vi "Change Voltage.vi"(8 "error in (no error)":errorcluster, 11 "Test Framework in":refnum<class "Test Framework.lvclass">) -> (0 "error out":errorcluster, 2 "PSU status":T1(array[cluster]), 3 "Test Framework out":refnum<class "Test Framework.lvclass">)   [LabVIEW 2020, in "Test Framework.lvclass"]
uses:
  Test Framework.lvclass
  Test Framework.lvclass/Test Framework.ctl
  Instruments/Power Supply/Power Supply.lvclass
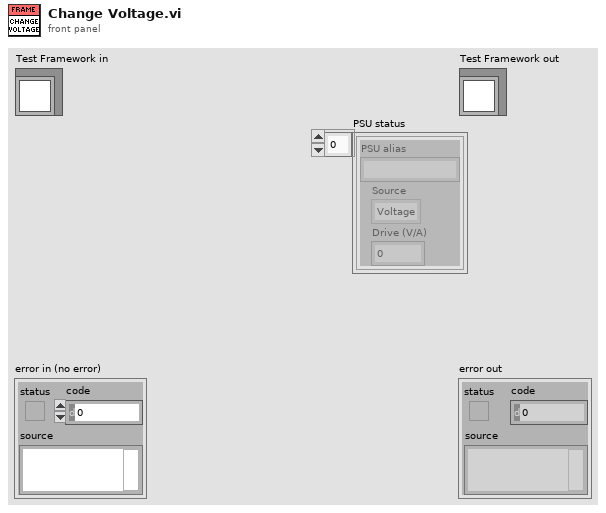
[diagram p1: front panel]
types:
  T1 = cluster{"PSU alias":string, "Source":enum32{"Voltage", "Current"}, "Drive (V/A)":dbl}[]
  T2 = cluster{"PSU alias":string, "Source":enum32{"Voltage", "Current"}, "Drive (V/A)":dbl}
  T3 = typedef "Test Framework.lvclass/Temperature and voltage array.ctl" = cluster{"Temperature [C]":dbl, "Soak time [m]":dbl, "PSUs":cluster{"Enabled":bool, "Source":enum32{"Voltage", "Current"}, "Drive (V/A)":dbl, "Sweep (V/A)":string, "Limit (A/V)":dbl, "PSU alias":string, "PSU info":cluster{"ID":string, "Address":string, "Channel":u8}}[]}[]
  T4 = typedef "Test Framework.lvclass/Temperature and voltage modes.ctl" = cluster{"Temperature mode":enum16{"Automatic", "Manual", "Off"}, "DC-Power mode":enum16{"Automatic", "Manual", "Off"}, "PSU sweep mode":bool, "Turn off after measurement":bool}
  T5 = cluster{"Temperature control array":T3, "Temperature mode":T4}
  T6 = cluster{"Temperature [C]":dbl, "Soak time [m]":dbl, "PSUs":cluster{"Enabled":bool, "Source":enum32{"Voltage", "Current"}, "Drive (V/A)":dbl, "Sweep (V/A)":string, "Limit (A/V)":dbl, "PSU alias":string, "PSU info":cluster{"ID":string, "Address":string, "Channel":u8}}[]}
  T7 = cluster{"Enabled":bool, "Source":enum32{"Voltage", "Current"}, "Drive (V/A)":dbl, "Sweep (V/A)":string, "Limit (A/V)":dbl, "PSU alias":string, "PSU info":cluster{"ID":string, "Address":string, "Channel":u8}}[]
  T8 = cluster{"ID":string, "Address":string, "Channel":u8}
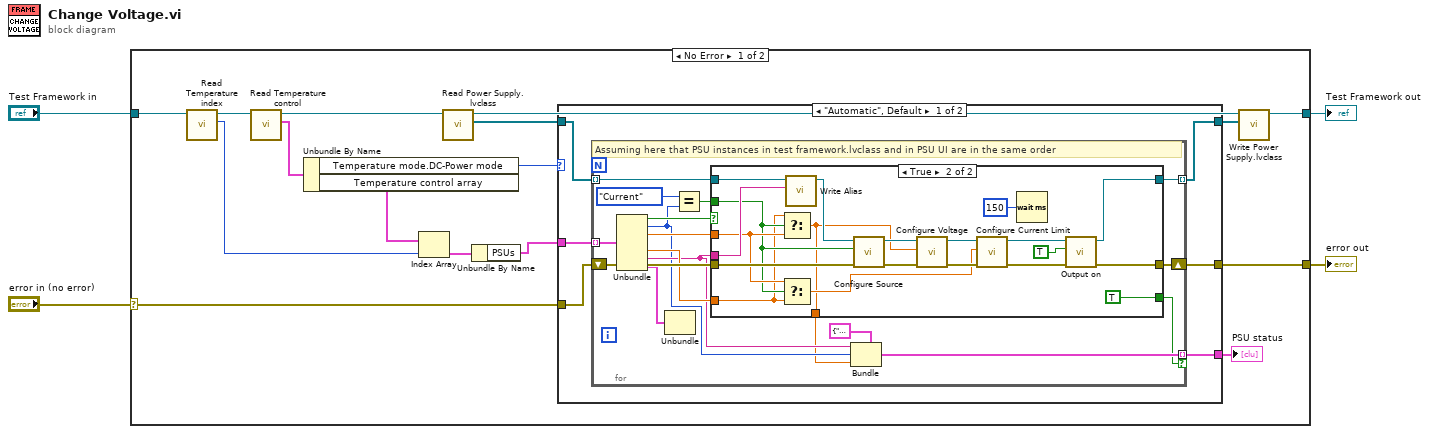
[diagram p0: block diagram]
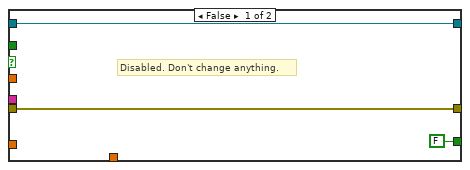
[diagram p2: hidden frame]
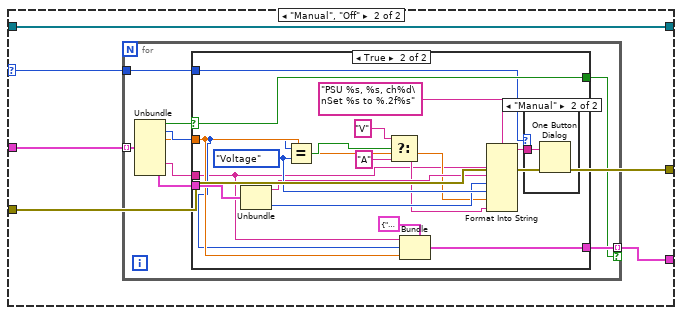
[diagram p3: hidden frame]
diagram:
  n1 = case shown="No Error" "error in (no error)" {
    selector: "error in (no error)" -> [w7 w100]
    tunnel: [w11 w100] -> w3
    tunnel: [w12 w99] -> w1
    tunnel: "Test Framework in" -> [w20 w99]
    frame No Error {
      n2 = call "Read Temperature index.vi"("Test Framework in"=w20) -> ("Environmental index"=w15:i32, "Test Framework out"=w19:refnum<class "Test Framework.lvclass">)  [unwired: 9 in]
      n3 = call-dynamic "Read Temperature control.vi"("Test Framework in"=w19) -> ("Temperature control"=w17:T5, "Test Framework out"=w18:refnum<class "Test Framework.lvclass">)  [unwired: 9 in]
      n4 = Unbundle By Name(w17) -> ("Temperature mode.DC-Power mode"=w8:enum16{"Automatic", "Manual", "Off"}, "Temperature control array"=w16:T3)
      n5 = Index Array(array=w16, index=w15) -> (element=w14:T6)
      n6 = call "Read Power Supply.lvclass.vi"("Test Framework in"=w18) -> ("Power Supply lvclasses"=w9:refnum<class "Power Supply.lvclass">[], "Test Framework out"=w13:refnum<class "Test Framework.lvclass">)  [unwired: 9 in]
      n7 = Unbundle By Name(w14) -> ("PSUs"=w6:T7)
      n8 = case shown="\"Automatic\", Default" w8 {
        selector: w8 -> [_ w68]
        tunnel: w9 -> [w26 w67]
        tunnel: [w25 w71] -> w11
        tunnel: w7 -> [w24 w71]
        tunnel: w6 -> [w23 w70]
        tunnel: [w22 w69] -> w5
        tunnel: [w21 w67] -> w10
        frame "Automatic", Default {
          n9 = for {
            shift-right: [w42] -> w25
            shift-left: w24 -> [w41]
            tunnel: w26 -> [w35] mode=indexing
            tunnel: [w43] -> w21 mode=indexing
            tunnel: w23 -> [w40] mode=indexing
            tunnel: [w29] -> w22 mode=indexing if=w28
            # "Assuming here that PSU instances in test framework.lvclass and in PSU UI are in the same order"
            n10 = Unbundle(w40) -> ("Enabled"=w38:bool, "Source"=w31:enum32{"Voltage", "Current"}, "Drive (V/A)"=w36:dbl, "Limit (A/V)"=w37:dbl, "PSU alias"=w32:string, "PSU info"=w39:T8)  [unwired: 1 out]
            n11 = Unbundle(w39) -> ()  [unwired: 3 out]
            n12 = Equal?(x=enum32{"Voltage", "Current"}."Current" ("Source"), y=w31) -> (x = y?=w33:bool)
            n13 = case shown="True" w38 {
              tunnel: w35 -> [w46 w56]
              tunnel: [w46 w66] -> w43
              tunnel: [w45 w65] -> w42
              tunnel: w41 -> [w45 w59]
              tunnel: w37 -> [_ w51]
              tunnel: w36 -> [_ w53]
              tunnel: w33 -> [_ w52]
              tunnel: w32 -> [_ w54]
              tunnel: [_ w49] -> w30
              tunnel: [FALSE TRUE] -> w28
              frame False {
                # "Disabled. Don't change anything."
              }
              frame True {
                n14 = Select(t=w51, s=w52, f=w53) -> (s? t:f=w49:dbl)
                n15 = Select(t=w53, s=w52, f=w51) -> (s? t:f=w50:dbl)
                n16 = call-dynamic "Write Alias.vi"("Alias"=w54, "Power Supply in"=w56) -> ("Power Supply out"=w55:refnum<class "Power Supply.lvclass">)  [unwired: 9 in]
                n17 = call-dynamic "Configure Source.vi"("error in (no error)"=w59, "Source (F:Volt)"=w52, "Power Supply in"=w55) -> ("error out"=w57:errorcluster, "Power Supply out"=w58:refnum<class "Power Supply.lvclass">)  [unwired: 7 in]
                n18 = call-dynamic "Configure Voltage.vi"("error in (no error)"=w57, "Voltage"=w49, "Power Supply in"=w58) -> ("error out"=w63:errorcluster, "Power Supply out"=w62:refnum<class "Power Supply.lvclass">)  [unwired: 7 in]
                n19 = call-dynamic "Configure Current Limit.vi"("error in (no error)"=w63, "Current Limit"=w50, "Power Supply in"=w62) -> ("error out"=w60:errorcluster, "Power Supply out"=w61:refnum<class "Power Supply.lvclass">)  [unwired: 7 in]
                n20 = Wait (ms)(milliseconds to wait=u32 150) -> ()  [unwired: 1 out]
                n21 = call-dynamic "Output on.vi"("error in (no error)"=w60, "Output On"=TRUE, "Power Supply in"=w61) -> ("error out"=w65:errorcluster, "Power Supply out"=w66:refnum<class "Power Supply.lvclass">)  [unwired: 7 in]
              }
            }
            n22 = Bundle(cluster=T2 {"PSU alias"="", "Source"=enum."Voltage", "Drive (V/A)"=0.0} ("PSU"), "PSU alias"=w32, "Source"=w31, "Drive (V/A)"=w30) -> (w29:T2)
          }
        }
        frame "Manual", "Off" {
          n23 = for {
            tunnel: w70 -> [w80] mode=indexing
            tunnel: [w74] -> w69 mode=indexing if=w73
            tunnel: w68 -> [w72]
            n24 = Unbundle(w80) -> ("Enabled"=w79:bool, "Source"=w78:enum32{"Voltage", "Current"}, "Drive (V/A)"=w77:dbl, "PSU alias"=w76:string, "PSU info"=w75:T8)  [unwired: 2 out]
            n25 = case shown="True" w79 {
              selector: w79 -> [_ w82]
              tunnel: w78 -> [_ w84]
              tunnel: w77 -> [_ w85]
              tunnel: w76 -> [_ w83]
              tunnel: w75 -> [_ w94]
              tunnel: [_ w86] -> w74
              tunnel: [_ w82] -> w73
              tunnel: w72 -> [_ w81]
              frame False {
              }
              frame True {
                w95 = enum32{"Voltage", "Current"}."Voltage" ("y")
                n26 = Unbundle(w94) -> ("ID"=w92:string, "Channel"=w93:u8)  [unwired: 1 out]
                n27 = Equal?(x=w84, y=w95) -> (x = y?=w89:bool)
                n28 = Select(t="V", s=w89, f="A") -> (s? t:f=w88:string)
                n29 = Bundle(cluster=T2 {"PSU alias"="", "Source"=enum."Voltage", "Drive (V/A)"=0.0} ("PSU"), "PSU alias"=w83, "Source"=w84, "Drive (V/A)"=w85) -> (w86:T2)
                n30 = Format Into String(format string="PSU %s, %s, ch%d\nSet %s to %.2f%s", w83, w92, w93, w95, w85, w88) -> (resulting string=w97:string)  [unwired: 2 in, 1 out]
                n31 = case shown="\"Manual\"" w81 {
                  tunnel: w97 -> [_ w98]
                  frame "Off", Default {
                  }
                  frame "Manual" {
                    n32 = One Button Dialog(message=w98) -> ()  [unwired: 1 in, 1 out]
                  }
                }
              }
            }
          }
        }
      }
      "PSU status" <- w5
      n33 = call "Write Power Supply.lvclass.vi"("Power Supply lvclasses"=w10, "Test Framework in"=w13) -> ("Test Framework out"=w12:refnum<class "Test Framework.lvclass">)  [unwired: 9 in]
    }
    frame Error {
    }
  }
  "error out" <- w3
  "Test Framework out" <- w1
